vi "Timing-Format Double Timestamp.vi"() -> ()   [LabVIEW 2020]
panel:
  out "date/time string":string
  in  "Numeric":dbl format="%#_20g"
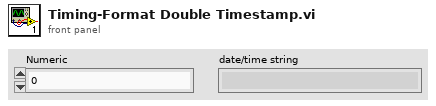
[diagram p1: front panel]
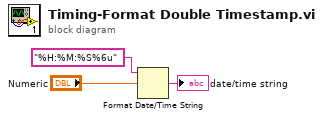
[diagram p0: block diagram]
diagram:
  n1 = Format Date/Time String(time format string (%c)="%H:%M:%S%6u", seconds (now)="Numeric") -> (date/time string=→"date/time string":string)  [unwired: 1 in]
